vi "first.vi"() -> ()   [LabVIEW 2019]
panel:
  out "Led":bool
  in  "button":bool
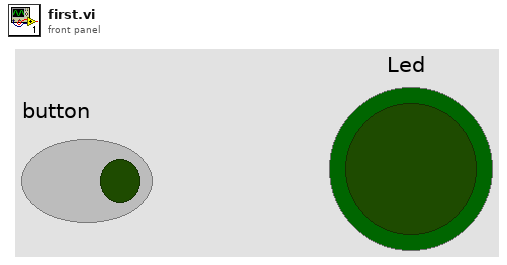
[diagram p1: front panel]
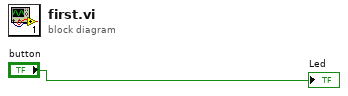
[diagram p0: block diagram]
diagram:
  "Led" <- "button"
